vi "ICM Calculate Time Stamps.vi"(6 "Second":dbl, 7 "Year":dbl, 8 "Minute":dbl, 9 "Hour":dbl, 10 "Day":dbl, 11 "Month":dbl) -> (2 "Seconds Since Midnight":dbl, 3 "TimeStamp":dbl)   [LabVIEW 2024]
doc: "ICM Calculate Time Stamps.vi\n\n This VI has the UTC date and time values as inputs and calculates the timestamps Seconds Since 1904 and Seconds Since Midnight.\n\nThis VI was original part of the OSDS system.\n\nInstrument Communication Module Version 1.0\nSeptember, 2017 Original Code Consulting David Thomson"
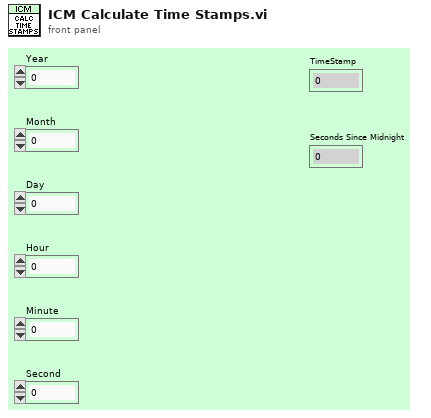
[diagram p1: front panel]
types:
  T1 = cluster{"fractional second":dbl, "second":i32, "minute":i32, "hour":i32, "day of month":i32, "month":i32, "year":i32, "day of week":i32, "day of year":i32, "DST":i32}
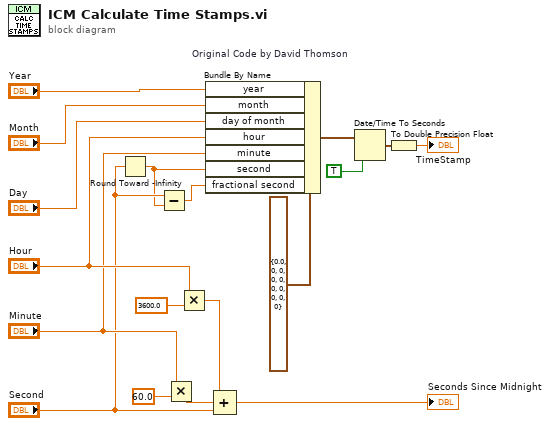
[diagram p0: block diagram]
diagram:
  w11 = T1 {"fractional second"=0.0, "second"=0, "minute"=0, "hour"=0, "day of month"=0, "month"=0, "year"=0, "day of week"=0, "day of year"=0, "DST"=0}  # Original Code by David Thomson
  n1 = Round Toward -Infinity(1:"Second") -> (0:w2:dbl)
  n2 = Subtract(x="Second", y=w2) -> (x-y=w1:dbl)
  n3 = Multiply(x="Minute", y=60.0) -> (x*y=w18:dbl)
  n4 = Multiply(x="Hour", y=3600.0) -> (x*y=w17:dbl)
  n5 = Bundle By Name(cluster=w11, "year"="Year", "month"="Month", "day of month"="Day", "hour"="Hour", "minute"="Minute", "second"=w2, "fractional second"=w1) -> (w14:T1)
  n6 = Compound Arithmetic op=ADD(w17, w18, "Second") -> (→"Seconds Since Midnight":dbl)
  n7 = Date/Time To Seconds(1:TRUE ("is UTC (F)"), 2:w14) -> (0:w12:timestamp)
  n8 = To Double Precision Float(number=w12) -> (double precision float=→"TimeStamp":dbl)
